vi "Writes_interdata.vi"(8 "error in (no error)":errorcluster, 10 "interdata":T1={"数据发送协议"=enum."2017-212协议", "枚举"=enum."返回请求应答", "系统编码ST"="21", "主动上报数据中"=FALSE, "数据组合发送"=FALSE, "地表水/污染源"=FALSE, "应用环境"=enum."STD"}, 11 "object in":refnum<class "212format_work.lvclass">) -> (0 "error out":errorcluster, 3 "object out":refnum<class "212format_work.lvclass">)   [LabVIEW 2016, in "212format_work.lvclass"]
uses:
  212format_work.lvclass
  212format_work.lvclass/212format_work.ctl
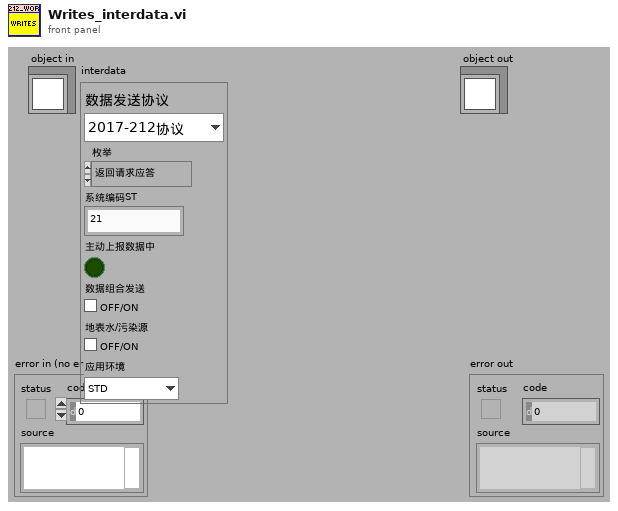
[diagram p1: front panel]
types:
  T1 = typedef "212format_work.lvclass/interdata控件.ctl" = cluster{"数据发送协议":enum16{"2005-212协议", "2017-212协议"}, "枚举":enum16{"返回请求应答", "上传数据", "返回执行结果"}, "系统编码ST":string, "主动上报数据中":bool, "数据组合发送":bool, "地表水/污染源":bool, "应用环境":enum16{"STD", "GB212"}}
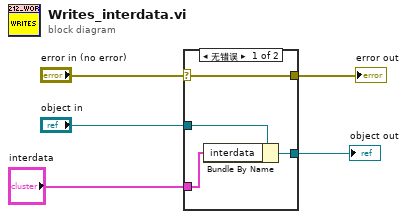
[diagram p0: block diagram]
diagram:
  n1 = case shown="无错误" "error in (no error)" {
    selector: "error in (no error)" -> [w9 w11]
    tunnel: [w9 w11] -> w4
    tunnel: [w7 w10] -> w2
    tunnel: "object in" -> [w8 w10]
    tunnel: "interdata" -> [w6 _]
    frame No Error {
      n2 = Bundle By Name(cluster=w8, "interdata"=w6) -> (w7:refnum<class "212format_work.lvclass">)
    }
    frame Error {
    }
  }
  "error out" <- w4
  "object out" <- w2
